vi "Write Enqueuer - Album Artwork.vi"(8 "error in (no error)":errorcluster, 10 "Actor Framework:Message Enqueuer":refnum<class "Message Enqueuer.lvclass">, 11 "SongQueueActor in":refnum<class "SongQueueActor.lvclass">) -> (0 "error out":errorcluster, 3 "SongQueueActor out":refnum<class "SongQueueActor.lvclass">)   [LabVIEW 2015, in "SongQueueActor.lvlib" / "SongQueueActor.lvclass"]
uses:
  SongQueueActor.lvclass
  <vilib>/ActorFramework/Message Enqueuer/Message Enqueuer.lvclass
  SongQueueActor.lvclass/SongQueueActor.ctl
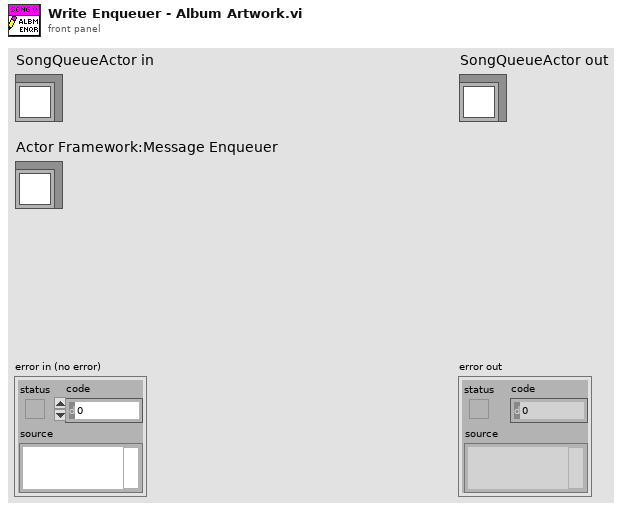
[diagram p1: front panel]
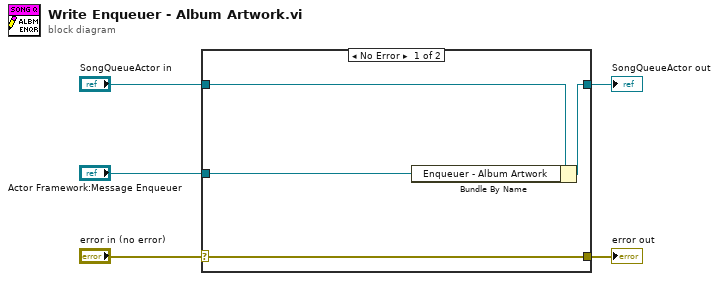
[diagram p0: block diagram]
diagram:
  n1 = case shown="No Error" "error in (no error)" {
    selector: "error in (no error)" -> [w9 w10]
    tunnel: [w9 w10] -> w4
    tunnel: [w7 w11] -> w2
    tunnel: "SongQueueActor in" -> [w8 w11]
    tunnel: "Actor Framework:Message Enqueuer" -> [w6 _]
    frame No Error {
      n2 = Bundle By Name(cluster=w8, "Enqueuer - Album Artwork"=w6) -> (w7:refnum<class "SongQueueActor.lvclass">)
    }
    frame Error {
    }
  }
  "error out" <- w4
  "SongQueueActor out" <- w2
